vi "get last register.vi"(11 "Modbus Module Channel in":refnum<class "Modbus Module Channel.lvclass">) -> (3 "last element":i32)   [LabVIEW 2013, in "Modbus Module Channel.lvclass"]
uses:
  Modbus Module Channel.lvclass
  <vilib>/NI/Tag Bus/tag/tag descriptor.lvclass/tag descriptor.ctl
  Modbus Module Channel.lvclass/Modbus Module Channel.ctl
  <vilib>/NI/Tag Bus/tag/tag descriptor.lvclass
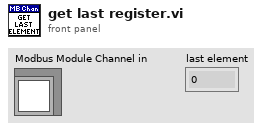
[diagram p1: front panel]
types:
  T1 = typedef "Modbus Module Channel.lvclass/data bank type.ctl" = enum16{"coils", "discrete inputs", "input registers", "holding registers"}
  T2 = typedef "tag bus.lvlib/tag descriptor.lvclass/Data Type.ctl" = enum16{"Double", "Single", "I64", "I32", "I16", "I8", "U64", "U32", "U16", "U8", "Boolean", "String", "Array of Double", "Array of Single", "Array of I64", "Array of I32", "Array of I16", "Array of I8", "Array of U64", "Array of U32", "Array of U16", "Array of U8", "Array of Boolean", "Array of String"}
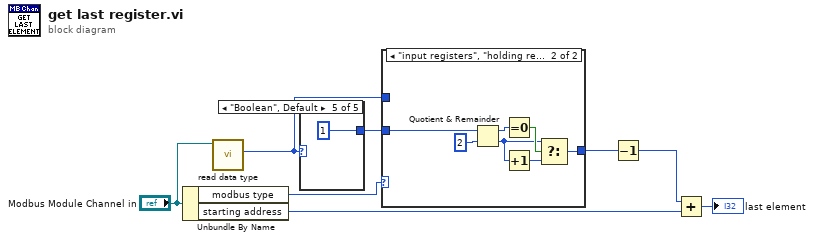
[diagram p0: block diagram]
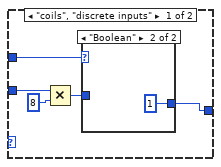
[diagram p2: hidden frame]
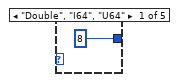
[diagram p4: hidden frame]
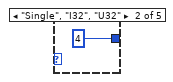
[diagram p5: hidden frame]
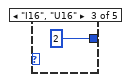
[diagram p6: hidden frame]
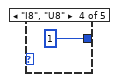
[diagram p7: hidden frame]
diagram:
  n1 = Unbundle By Name("Modbus Module Channel in") -> ("modbus type"=w4:T1, "starting address"=w8:u16)
  n2 = call <vilib>:"read data type.vi"("system tag in"="Modbus Module Channel in") -> ("data type"=w2:T2)  [unwired: 8 in, 2 out]
  n3 = case shown="\"Boolean\", Default" w2 {
    tunnel: [8 ("x") 4 ("x") 2 ("x") 1 ("x") 1 ("x")] -> w5
    frame "Double", "I64", "U64" {
    }
    frame "Single", "I32", "U32" {
    }
    frame "I16", "U16" {
    }
    frame "I8", "U8" {
    }
    frame "Boolean", Default {
    }
  }
  n4 = case shown="\"input registers\", \"holding registers\"" w4 {
    tunnel: w5 -> [w18 w27]
    tunnel: [w15 w21] -> w3
    tunnel: w2 -> [w16 _]
    frame "coils", "discrete inputs" {
      n5 = Multiply(x=w18, y=8) -> (x*y=w14:i32)
      n6 = case shown="\"Boolean\"" w16 {
        tunnel: [w19 1] -> w15
        tunnel: w14 -> [w19 _]
        frame Default {
        }
        frame "Boolean" {
        }
      }
    }
    frame "input registers", "holding registers" {
      n7 = Quotient & Remainder(x=w27, y=2) -> (x-y*floor(x/y)=w25:i32, floor(x/y)=w23:i32)
      n8 = Equal To 0?(x=w25) -> (x = 0?=w24:bool)
      n9 = Increment(x=w23) -> (x+1=w22:i32)
      n10 = Select(t=w23, s=w24, f=w22) -> (s? t:f=w21:i32)
    }
  }
  n11 = Decrement(x=w3) -> (x-1=w1:i32)
  n12 = Add(x=w1, y=w8) -> (x+y=→"last element":i32)
